vi "Update Core.vi"(8 "error in (no error)":errorcluster, 11 "Dual Fan in":refnum<class "Dual Fan.lvclass">) -> (0 "error out":errorcluster, 3 "Dual Fan out":refnum<class "Dual Fan.lvclass">)   [LabVIEW 2025, in "Dual Fan.lvlib" / "Dual Fan.lvclass"]
doc: "Every poll interval, check for a hardware fail and switch fans as needed."
uses:
  Dual Fan.lvclass
  Fan Info.ctl
  Dual Fan.lvclass/Dual Fan.ctl
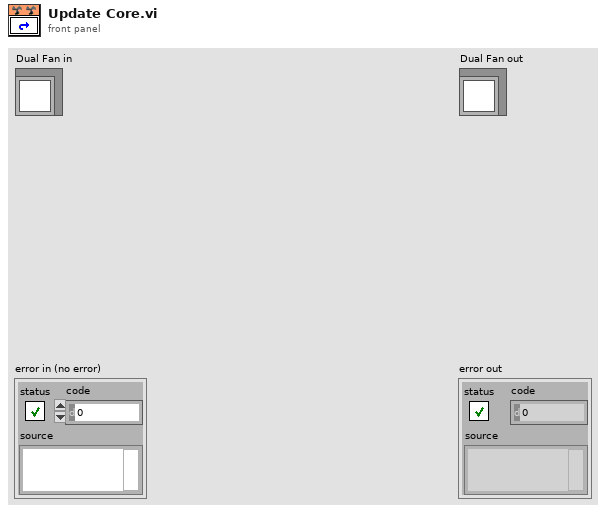
[diagram p1: front panel]
types:
  T1 = typedef "Dual Fan.lvlib/Dual Fan.lvclass/Fan Info.ctl" = cluster{"State":bool, "Fault":bool}
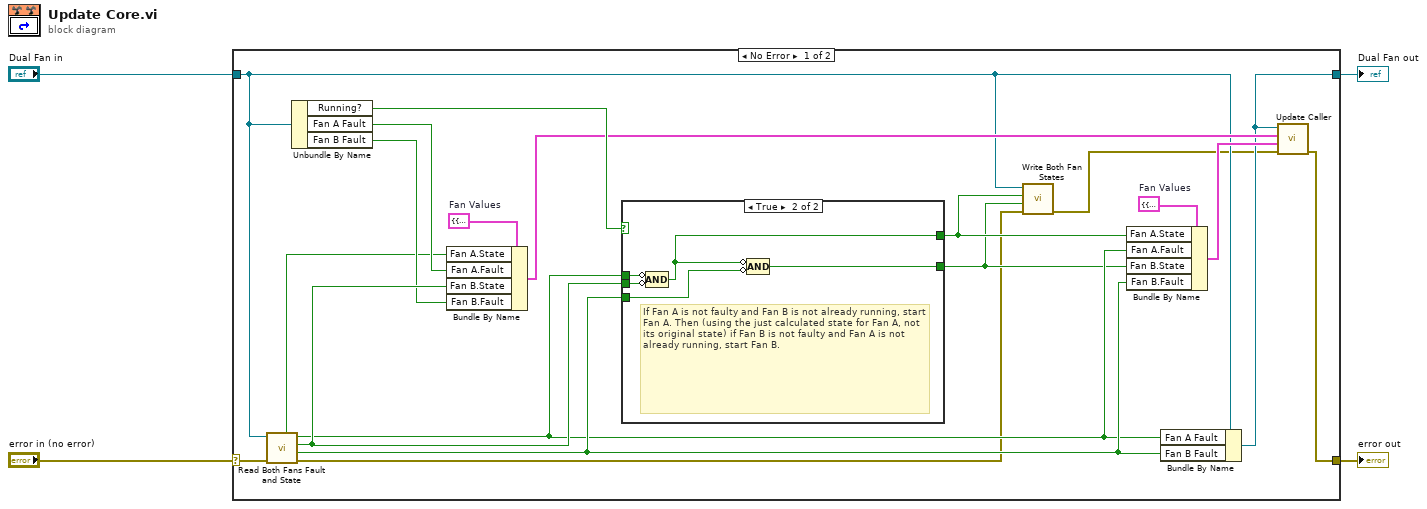
[diagram p0: block diagram]
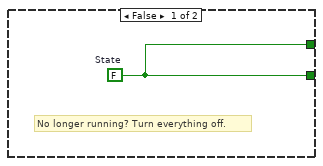
[diagram p2: hidden frame]
diagram:
  n1 = case shown="No Error" "error in (no error)" {
    selector: "error in (no error)" -> [w15 w31]
    tunnel: [w23 w31] -> w3
    tunnel: [w16 w30] -> w1
    tunnel: "Dual Fan in" -> [w9 w30]
    frame No Error {
      w13 = cluster{"Fan A":T1, "Fan B":T1} {"Fan A"={"State"=FALSE, "Fault"=FALSE}, "Fan B"={"State"=FALSE, "Fault"=FALSE}}  # Fan Values
      w14 = cluster{"Fan A":T1, "Fan B":T1} {"Fan A"={"State"=FALSE, "Fault"=FALSE}, "Fan B"={"State"=FALSE, "Fault"=FALSE}}  # Fan Values
      n2 = call-dynamic "Read Both Fans Fault and State.vi"("error in (no error)"=w15, "Dual Fan in"=w9) -> ("error out"=w5:errorcluster, "Fan B Fault"=w11:bool, "Fan B State"=w21:bool, "Fan A Fault"=w10:bool, "Fan A State"=w12:bool)  [unwired: 5 in]
      n3 = Unbundle By Name(w9) -> ("Running?"=w22:bool, "Fan A Fault"=w20:bool, "Fan B Fault"=w19:bool)
      n4 = Bundle By Name(cluster=w13, "Fan A.State"=w12, "Fan A.Fault"=w20, "Fan B.State"=w21, "Fan B.Fault"=w19) -> (w17:cluster{"Fan A":T1, "Fan B":T1})
      n5 = case shown="True" w22 {
        tunnel: w21 -> [_ w27]
        tunnel: w10 -> [_ w29]
        tunnel: w11 -> [_ w28]
        tunnel: [w24 w26] -> w8
        tunnel: [w24 w25] -> w7
        frame False {
          w24 = FALSE  # State
          # "No longer running? Turn everything off."
        }
        frame True {
          # "If Fan A is not faulty and Fan B is not already running, start Fan A. Then (using the just calculated state for Fan A, not its original state) if Fan B is not faulty and Fan A is not already running, start Fan B."
          n6 = Compound Arithmetic op=AND(invert w29, invert w27) -> (w26:bool)
          n7 = Compound Arithmetic op=AND(invert w26, invert w28) -> (w25:bool)
        }
      }
      n8 = call-dynamic "Write Both Fan States.vi"("error in (no error)"=w5, "Fan B State"=w7, "Fan A State"=w8, "Dual Fan in"=w9) -> ("error out"=w6:errorcluster)  [unwired: 7 in]
      n9 = Bundle By Name(cluster=w14, "Fan A.State"=w8, "Fan A.Fault"=w10, "Fan B.State"=w7, "Fan B.Fault"=w11) -> (w18:cluster{"Fan A":T1, "Fan B":T1})
      n10 = Bundle By Name(cluster=w9, "Fan A Fault"=w10, "Fan B Fault"=w11) -> (w16:refnum<class "Dual Fan.lvclass">)
      n11 = call "Update Caller.vi"("error in (no error)"=w6, "New Values"=w18, "Old Values"=w17, "Dual Fan"=w16) -> ("error out"=w23:errorcluster)  [unwired: 7 in]
    }
    frame Error {
    }
  }
  "error out" <- w3
  "Dual Fan out" <- w1
